vi "Measure_Temp_Sensor.vi"(8 "error in (no error)":errorcluster, 10 "Parameters":string, 11 "reference in":refnum<class "Test_Flux_Capacitor.lvclass">) -> (0 "error out":errorcluster, 2 "Result":i32, 3 "reference out":refnum<class "Test_Flux_Capacitor.lvclass">)   [LabVIEW 2022 SP3, in "Test_Flux_Capacitor.lvlib" / "Test_Flux_Capacitor.lvclass"]
uses:
  Test_Flux_Capacitor.lvclass
  ParameterTypes/TempSensor.ctl
  Components/SwitchBase.lvlibp/SwitchBase.lvclass
  Components/PSU_Base.lvlibp/PSU_Base.lvclass
  <vilib>/JDP Science/JSONtext/JSONtext.lvlib
panel:
  in  "Parameter_Type":T1
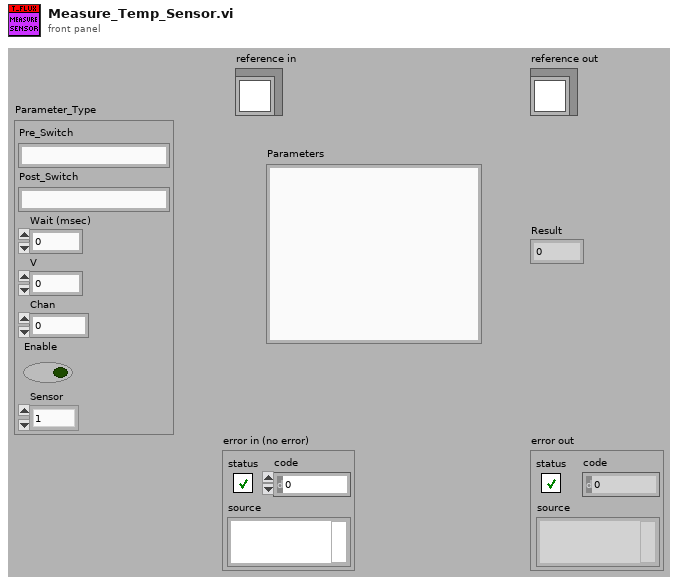
[diagram p1: front panel]
types:
  T1 = typedef "Test_Flux_Capacitor.lvlib/Test_Flux_Capacitor.lvclass/TempSensor.ctl" = cluster{"Pre_Switch":string, "Post_Switch":string, "Wait (msec)":u32, "V":dbl, "Chan":i32, "Enable":bool, "Sensor":enum16{"1", "2", "3"}}
  T2 = typedef "Test_Flux_Capacitor.lvlib/Test_Flux_Capacitor.lvclass/ObjectAttributes.ctl" = cluster{"Config":T3, "DMM":refnum<class "DMM_Keysight_34980A.lvclass">, "LCR":refnum<class "LCR_BK891.lvclass">, "PSU":refnum<class "PSU_Base.lvclass">, "Switch_Manager":refnum<class "SwitchBase.lvclass">, "FRAM":string, "Flux_Capacitor":refnum<class "Flux_Capacitor.lvclass">, "Frequency_Counter":refnum<class "Frequency_Counter_Base.lvclass">, "JTAG":refnum<class "JTAG_Base.lvclass">}
  T3 = typedef "Test_Flux_Capacitor.lvlib/Test_Flux_Capacitor.lvclass/Config.ctl" = cluster{"default":string}
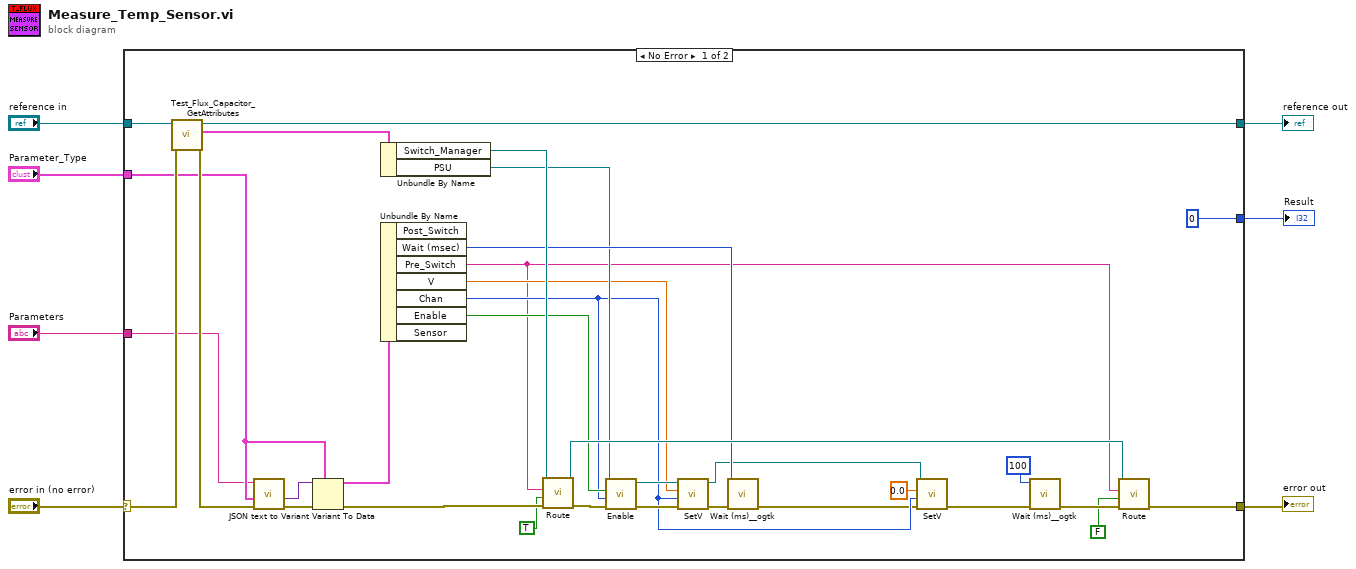
[diagram p0: block diagram]
diagram:
  n1 = case shown="No Error" "error in (no error)" {
    selector: "error in (no error)" -> [w40 w42]
    tunnel: [w33 w42] -> w6
    tunnel: [w38 w41] -> w4
    tunnel: "reference in" -> [w39 w41]
    tunnel: "Parameters" -> [w14 _]
    tunnel: "Parameter_Type" -> [w15 _]
    tunnel: [0 _] -> w1
    frame No Error {
      n2 = call "Test_Flux_Capacitor_GetAttributes.vi"("error in (no error)"=w40, "reference in"=w39) -> ("error out"=w17:errorcluster, "Data"=w37:T2, "reference out"=w38:refnum<class "Test_Flux_Capacitor.lvclass">)  [unwired: 6 in, 1 out]
      n3 = call <vilib>:"JSON text to Variant.vi"("error in (no error)"=w17, "Data Type"=w15, "JSON"=w14) -> ("error out"=w16:errorcluster, "Variant out"=w13:variant)  [unwired: 7 in]
      n4 = Variant To Data(error in=w16, type=w15, Variant=w13) -> (data=w36:T1, error out=w32:errorcluster)
      n5 = Unbundle By Name(w37) -> ("Switch_Manager"=w35:refnum<class "SwitchBase.lvclass">, "PSU"=w27:refnum<class "PSU_Base.lvclass">)
      n6 = Unbundle By Name(w36) -> ("Wait (msec)"=w31:u32, "Pre_Switch"=w11:string, "V"=w24:dbl, "Chan"=w19:i32, "Enable"=w25:bool)  [unwired: 2 out]
      n7 = call-dynamic "Route.vi"("error in (no error)"=w32, "Connect"=TRUE, "channel 1"=w11, "reference in"=w35) -> ("error out"=w30:errorcluster, "reference in"=w34:refnum<class "SwitchBase.lvclass">)  [unwired: 6 in]
      n8 = call-dynamic "Enable.vi"("error in (no error)"=w30, "Chan"=w19, "Enable"=w25, "reference in"=w27) -> ("error out"=w29:errorcluster, "reference in"=w26:refnum<class "PSU_Base.lvclass">)  [unwired: 6 in]
      n9 = call-dynamic "SetV.vi"("error in (no error)"=w29, "Chan"=w19, "V"=w24, "reference in"=w26) -> ("error out"=w28:errorcluster, "reference in"=w23:refnum<class "PSU_Base.lvclass">)  [unwired: 6 in]
      n10 = call <userlib>:"Wait (ms)__ogtk.vi"("error in (no error)"=w28, "milliseconds to wait"=w31) -> ("error out"=w9:errorcluster)  [unwired: 8 in, 1 out]
      n11 = call-dynamic "SetV.vi"("error in (no error)"=w9, "Chan"=w19, "V"=0.0, "reference in"=w23) -> ("error out"=w18:errorcluster)  [unwired: 6 in, 1 out]
      n12 = call <userlib>:"Wait (ms)__ogtk.vi"("error in (no error)"=w18, "milliseconds to wait"=u32 100) -> ("error out"=w21:errorcluster)  [unwired: 8 in, 1 out]
      n13 = call-dynamic "Route.vi"("error in (no error)"=w21, "Connect"=FALSE, "channel 1"=w11, "reference in"=w34) -> ("error out"=w33:errorcluster)  [unwired: 6 in, 1 out]
    }
    frame Error {
    }
  }
  "Result" <- w1
  "error out" <- w6
  "reference out" <- w4
